vi "FTW-Container-QueryValue.vi"(0 "Container":refnum<class "FTW-Container.lvclass">, 5 "Type and Defaults":variant, 11 "error in":errorcluster) -> (4 "Container out":refnum<class "FTW-Container.lvclass">, 6 "Result":variant, 15 "error out":errorcluster)   [LabVIEW 2012, in "FTW-Container.lvclass"]
uses:
  FTW-Container.lvclass
  JSON/FTW-JSON-RegexParse.vi
  Regex/FTW-Regex.vi
  JSON/FTW-JSON-RegexHeader.vi
  Error/FTW-ERR-ThrowError.vi
  Error/FTW-ERR-ThrowGenericError.vi
  FTW-Container-Construct.vi
  FTW-Container-Load-JSON.vi
  FTW-Container-Destroy.vi
  JSON/FTW-JSON-Deserialize.xnode
panel:
  # "Inputs"
  # "Outputs"
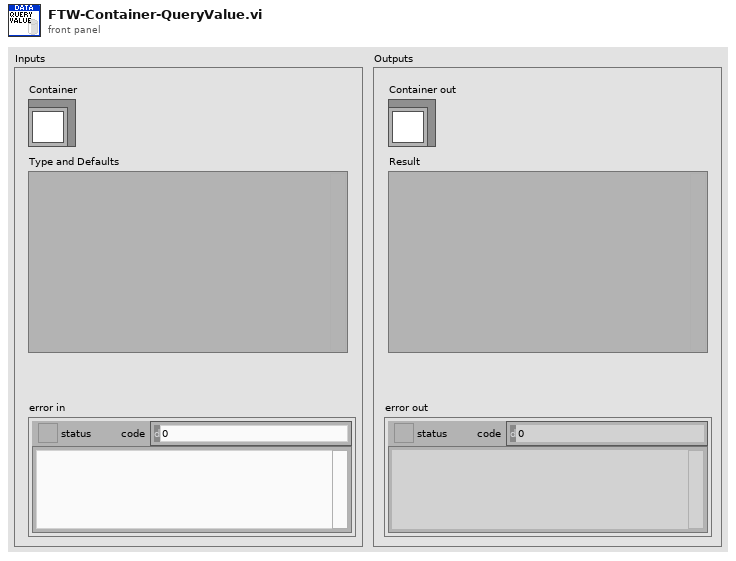
[diagram p1: front panel]
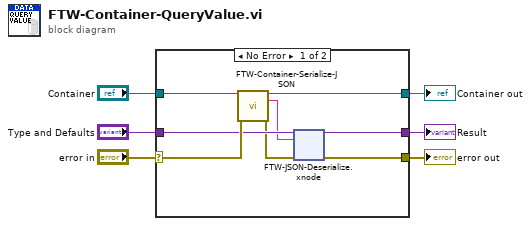
[diagram p0: block diagram]
diagram:
  n1 = case shown="No Error" "error in" {
    selector: "error in" -> [w12 w50]
    tunnel: [w8 w50] -> w6
    tunnel: "Container" -> [w14 w49]
    tunnel: [w13 w49] -> w3
    tunnel: "Type and Defaults" -> [w11 w48]
    tunnel: [w7 w48] -> w1
    frame No Error {
      n2 = call "FTW-Container-Serialize-JSON.vi"("Container"=w14, "error in"=w12) -> ("Container out"=w13:refnum<class "FTW-Container.lvclass">, "Serialized Container"=w10:string, "error out"=w9:errorcluster)  [unwired: 11 in]
      n3 = xnode "FTW-JSON-Deserialize.xnode"("Data Type and Default Values"=w11, "JSON String"=w10, "error in"=w9) -> ("Populated Values"=w7:variant, "error out"=w8:errorcluster)
    }
    frame Error {
    }
  }
  "error out" <- w6
  "Container out" <- w3
  "Result" <- w1
